vi "Max-iteration.vi"(0 "i max":i32, 2 "i act":i32, 3 "Valeur entrante":bool) -> (1 "break ?":bool)   [LabVIEW 2011]
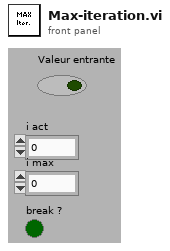
[diagram p1: front panel]
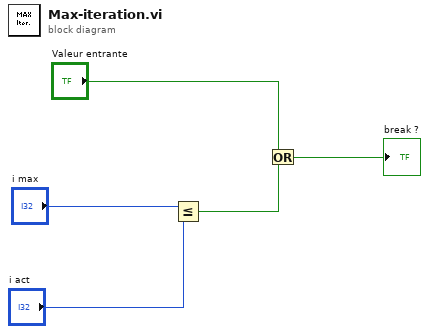
[diagram p0: block diagram]
diagram:
  n1 = Less Or Equal?(x="i max", y="i act") -> (x <= y?=w3:bool)
  n2 = Or(x="Valeur entrante", y=w3) -> (x .or. y?=→"break ?":bool)
